vi "数组数据运算-加法.vi"() -> ()   [LabVIEW 2014]
panel:
  out "结果 3":dbl[][](array[numeric])
  in  "数组 2":dbl[][](array[numeric])
  in  "数组1":dbl[][](array[numeric])
  out "结果 2":dbl[](array[numeric])
  out "结果":dbl[](array[numeric])
  in  "数值":dbl=4.0
  in  "数组b":dbl[](array[numeric])
  in  "数组a":dbl[](array[numeric])
  in  "数组":dbl[](array[numeric])=[1.0, 2.0, 3.0]
  # "+"
  # "="
  # "+"
  # "="
  # "+"
  # "="
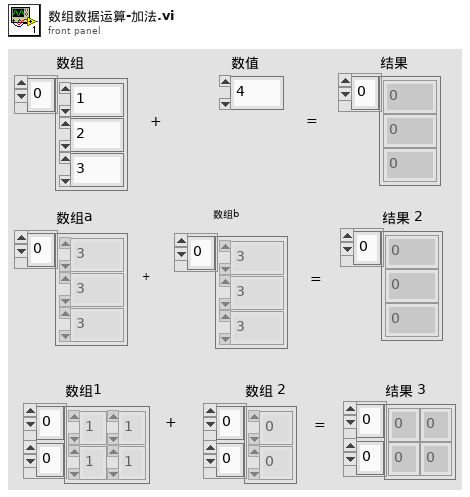
[diagram p1: front panel]
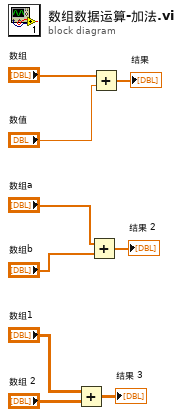
[diagram p0: block diagram]
diagram:
  n1 = Add(x="数组1", y="数组 2") -> (x+y=→"结果 3":dbl[][])
  n2 = Add(x="数组a", y="数组b") -> (x+y=→"结果 2":dbl[])
  n3 = Add(x="数组", y="数值") -> (x+y=→"结果":dbl[])
